vi "Execute Linear Output - Adding Points.vi"() -> ()   [LabVIEW 2017]
doc: "This VI is the host VI for the Linear Output - Adding Points VI. It sets the control values for the VI, then it executes the VI, which has been downloaded to an FPGA."
uses:
  <vilib>/rvi/interface/nirviCloseFPGA/nirviCloseFPGA.xnode
  <vilib>/rvi/interface/nirviMethod/nirviMethod.xnode
  <vilib>/rvi/interface/nirviReadWriteControl/nirviReadWriteControl.xnode
  <vilib>/rvi/interface/nirviOpenFPGA/nirviOpenFPGA.xnode
  Linear Output - Adding Points (FPGA).vi
  <vilib>/rvi/interface/RandomDataEmulation/nirviRandomDataOpen.vi
  <vilib>/rvi/interface/RandomDataEmulation/niFpgaWriteControlTemplate.vi
  <vilib>/rvi/interface/RandomDataEmulation/nirviRandomDataRunMethod.vi
  <vilib>/rvi/interface/RandomDataEmulation/nirviRandomDataClose.vi
panel:
  out "error out":errorcluster
  in  "resource name":refnum<visa-resource-name>="RIO0::INSTR"
  in  "Update Period (mSec)":u32=500
  in  "End Point":i16=32767
  in  "Start Point":i16=-32768
  in  "Points to Add (2^n - 1)":i16=3
  # "* The Linear Output - Adding Points VI will output voltages between the Start Point\nand End Point values.  The number of points that  will be placed is determined by the \nPoints to Add control, and they will be output at a rate equal to 1/Update Period (mSec)"
  # "* The number of points to add will equal:  2^(Points To Add) - 1;"
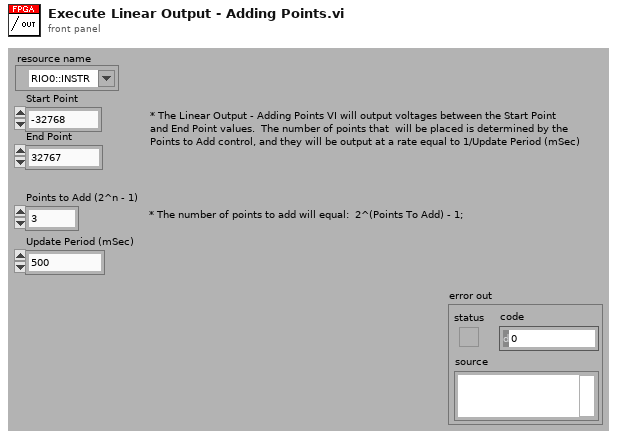
[diagram p1: front panel]
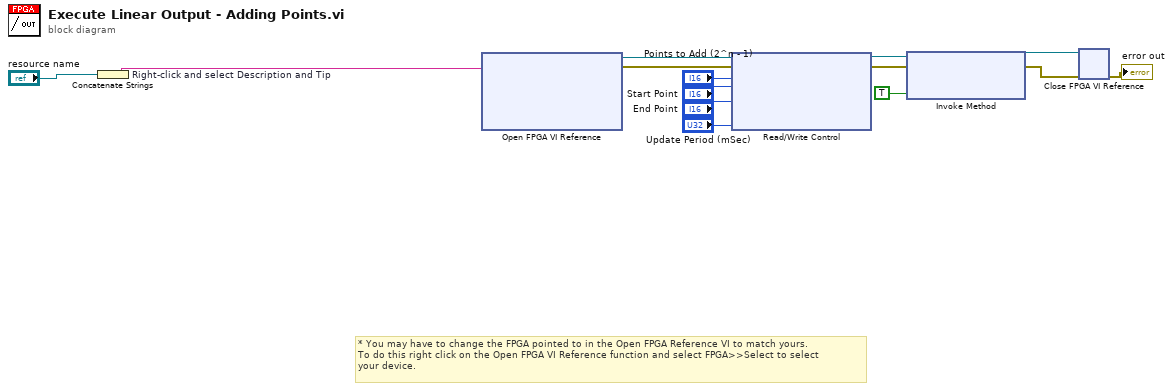
[diagram p0: block diagram]
diagram:
  # "* You may have to change the FPGA pointed to in the Open FPGA Reference VI to match yours.\nTo do this right click on the Open FPGA VI Reference function and select FPGA>>Select to select\nyour device."
  n1 = Concatenate Strings "Right-click and select Description and Tip"("resource name") -> (w1:string)
  n2 = xnode "Open FPGA VI Reference"("resource name"=w1) -> ("FPGA VI Reference Out"=w13:refnum<k20>, "error out"=w14:errorcluster)  [unwired: 1 in]
  n3 = xnode "Read/Write Control"("FPGA VI Reference In"=w13, "error in"=w14, "Points to Add (2^n - 1)"="Points to Add (2^n - 1)", "Start Point"="Start Point", "End Point"="End Point", "Update Period (mSec)"="Update Period (mSec)") -> ("FPGA VI Reference Out"=w8:refnum<k20>, "error out"=w7:errorcluster)
  n4 = xnode "Invoke Method"("FPGA VI Reference In"=w8, "error in"=w7, "Wait Until Done (F)"=TRUE) -> ("FPGA VI Reference Out"=w6:refnum<k20>, "error out"=w5:errorcluster)
  n5 = xnode "Close FPGA VI Reference"("FPGA VI Reference In"=w6, "error in"=w5) -> ("error out"=→"error out":errorcluster)
